vi "Initialize Front Panel.vi"(8 "error in (no error)":errorcluster, 11 "IViewable in":refnum<class "IViewable.lvclass">) -> (0 "error out":errorcluster, 3 "IViewable out":refnum<class "IViewable.lvclass">)   [LabVIEW 2020, in "IViewable.lvlib" / "IViewable.lvclass"]
doc: "初始化前面板"
uses:
  IViewable.lvclass
  IViewable.lvclass/IViewable.ctl
  ApplicationStyleReference/ApplicationStyleReference.lvclass/ApplicationStyleReference.ctl
  IApplicationStyle/IApplicationStyle.lvclass
  ApplicationStyleReference/ApplicationStyleReference.lvclass
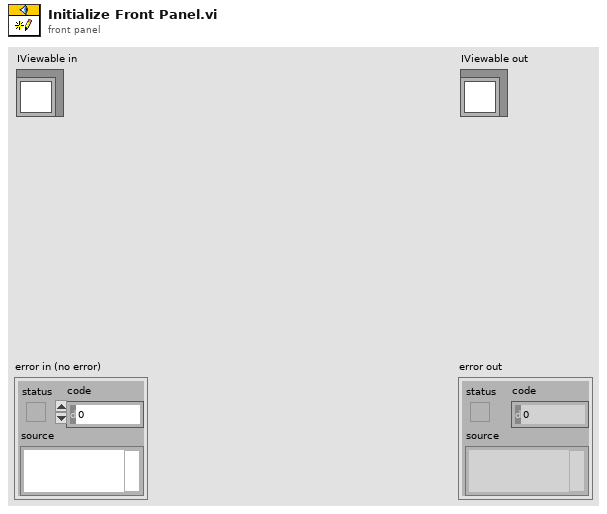
[diagram p1: front panel]
types:
  T1 = typedef "IViewable.lvlib/ApplicationStyleReference.lvclass/Application Style Reference.ctl" = refnum<data-value>
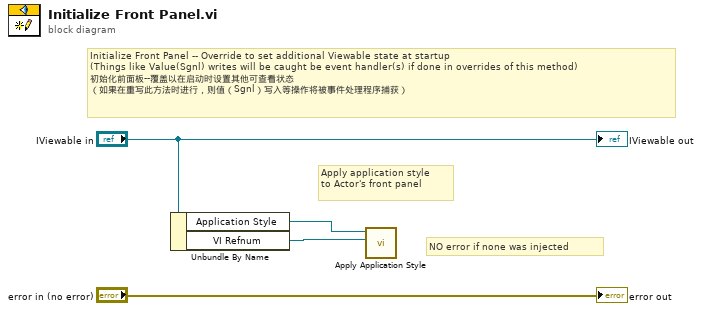
[diagram p0: block diagram]
diagram:
  # "NO error if none was injected"
  # "Apply application style\nto Actor's front panel"
  # "Initialize Front Panel -- Override to set additional Viewable state at startup\n(Things like Value(Sgnl) writes will be caught be event handler(s) if done in overrides of this method)\n初始化前面板--覆盖以在启动时设置其他可查看状态\n（如果在重写此方法时进行，则值（Sgnl）写入等操作将被事件处理程序捕获）"
  n1 = Unbundle By Name("IViewable in") -> ("Application Style"=w3:T1, "VI Refnum"=w2:refnum<vi>)
  n2 = call "Apply Application Style.vi"("VI Refnum"=w2, "ApplicationStyleReference in"=w3) -> ()  [unwired: 9 in, 1 out]
  "error out" <- "error in (no error)"
  "IViewable out" <- "IViewable in"
